vi "Test_playback_indicator.vi"() -> ()   [LabVIEW 2018]
panel:
  in  "Numeric 3":dbl format="%#_13g"
  in  "Numeric 2":dbl format="%#_13g"
  in  "Numeric":dbl format="%#_13g"
  in  "Timeline":T1(slide)={"Slider"=0.0, "Slider"=648.2670807453416, "Slider"=2749.5465838509317} scale=0.0..3599.0 scale format="%<%H:%M:%S>t"
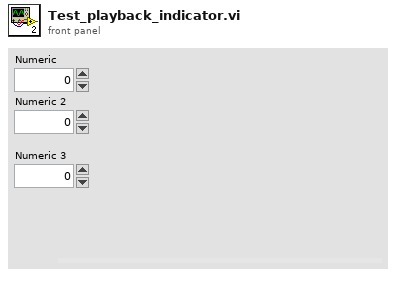
[diagram p1: front panel]
types:
  T1 = cluster{"Slider":dbl, "Slider":dbl, "Slider":dbl}
  T2 = cluster{"Numeric":dbl, "Numeric 2":dbl, "Numeric 3":dbl}
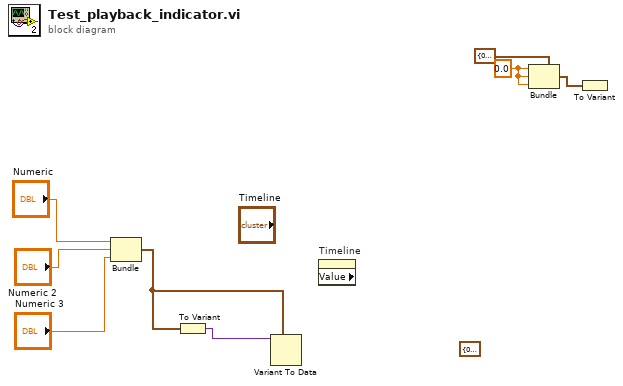
[diagram p0: block diagram]
diagram:
  w1 = 0.0 ("Slider")
  (unwired) T1 {"Slider"=0.0, "Slider"=0.0, "Slider"=0.0} ("Timeline")
  n1 = Bundle("Numeric"="Numeric", "Numeric 2"="Numeric 2", "Numeric 3"="Numeric 3") -> (w4:T2)  [unwired: 1 in]
  n2 = To Variant(anything=w4) -> (Variant=w5:variant)
  n3 = Variant To Data(type=w4, Variant=w5) -> ()  [unwired: 1 in, 2 out]
  n4 = property on="Timeline" class="Slide (strict)" props=["Value"]() -> ()  [unwired: 2 in, 3 out]
  n5 = Bundle(cluster=T1 {"Slider"=0.0, "Slider"=0.0, "Slider"=0.0} ("Timeline"), "Slider"=w1, "Slider"=w1, "Slider"=w1) -> (w2:T1)
  n6 = To Variant(anything=w2) -> ()  [unwired: 1 out]
